vi "Position_Based_Vacuum_Force.vi"(8 "vac_bnd":dbl[](array[numeric])=[80.0, 100.0], 9 "z_thld":dbl[](array[numeric])=[0.5, 2.5], 10 "current zp":dbl, 11 "current z":dbl) -> (3 "vacf (%)":dbl)   [LabVIEW 2010]
doc: "This VI calculates the vacuum force based on the distance to posterior capsule.\nDistance to posterior capsule is calculated by (current z) - (current zp)\nThe vacuum force is scheduled with some threshold values:\nif z_dist < z_thld(0), vacf = vac_bnd(0);\nif z_dist > z_thld(1), vacf = vac_bnd(1);\nif z_dist is somewhere in between, it propagates linearly."
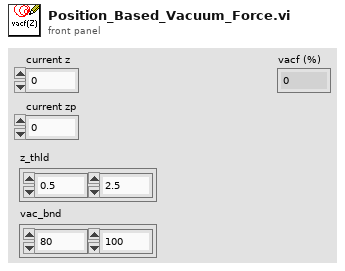
[diagram p1: front panel]
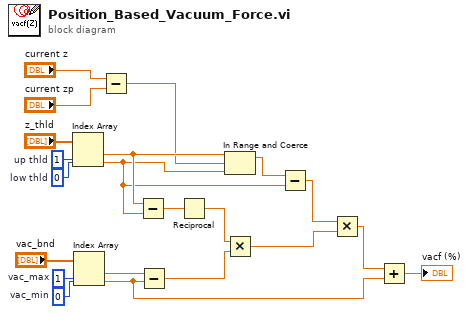
[diagram p0: block diagram]
diagram:
  w16 = 0  # vac_min
  w17 = 1  # vac_max
  w19 = 0  # low thld
  w20 = 1  # up thld
  n1 = Index Array(array="z_thld", index #1=w20, index #2=w19) -> (element #1=w15:dbl, element #2=w9:dbl)
  n2 = Index Array(array="vac_bnd", index #1=w17, index #2=w16) -> (element #1=w14:dbl, element #2=w8:dbl)
  n3 = Subtract(x="current z", y="current zp") -> (x-y=w1:dbl)
  n4 = Subtract(x=w15, y=w9) -> (x-y=w13:dbl)
  n5 = Subtract(x=w14, y=w8) -> (x-y=w11:dbl)
  n6 = Reciprocal(x=w13) -> (1/x=w12:dbl)
  n7 = In Range and Coerce(upper limit=w15, x=w1, lower limit=w9) -> (coerced(x)=w10:dbl)  [unwired: 1 out]
  n8 = Multiply(x=w12, y=w11) -> (x*y=w6:dbl)
  n9 = Subtract(x=w10, y=w9) -> (x-y=w7:dbl)
  n10 = Multiply(x=w7, y=w6) -> (x*y=w5:dbl)
  n11 = Add(x=w5, y=w8) -> (x+y=→"vacf (%)":dbl)
